vi "run_test_item.vi"(7 "DAQmx Device Name":tag="Dev1", 8 "error in":errorcluster, 10 "Test item":T2) -> (0 "error out":errorcluster, 1 "Test result":T1, 2 "Cluster":T6 {"Time Stamp" format="%<%.3X>T"})   [LabVIEW 2024]
doc: "The VI's input is a ctl_test_item_cluster. The output is the ctl_results_cluster indicator:\n- Time stamp: is the current time\n- Test item name: is the same as the Test item control's same label\n- Efficiency, Input Voltage, Output Voltage: pass criteria fulfilment for the measurement performed (perfrom_measurement.vi) based on the Test item.Stimuli cluster, results compared to the Test item.Pass limits cluster"
uses:
  OneDrive - Aalto University/SSIs - Semester 3/BME (1)/BME/vim report/dcdc_validator_project_Final (2)/dcdc_validator_project_Final/ctl_results_cluster.ctl
  OneDrive - Aalto University/SSIs - Semester 3/BME (1)/BME/vim report/dcdc_validator_project_Final (2)/dcdc_validator_project_Final/ctl_pass_fail_led.ctl
  OneDrive - Aalto University/SSIs - Semester 3/BME (1)/BME/vim report/dcdc_validator_project_Final (2)/dcdc_validator_project_Final/ctl_test_item_cluster.ctl
  OneDrive - Aalto University/SSIs - Semester 3/BME (1)/BME/vim report/dcdc_validator_project_Final (2)/dcdc_validator_project_Final/ctl_stimuli_cluster.ctl
  OneDrive - Aalto University/SSIs - Semester 3/BME (1)/BME/vim report/dcdc_validator_project_Final (2)/dcdc_validator_project_Final/ctl_loads_enum.ctl
  OneDrive - Aalto University/SSIs - Semester 3/BME (1)/BME/vim report/dcdc_validator_project_Final (2)/dcdc_validator_project_Final/ctl_pass_limits_cluster.ctl
  OneDrive - Aalto University/SSIs - Semester 3/BME (1)/BME/vim report/dcdc_validator_project_Final (2)/dcdc_validator_project_Final/ctl_test_outputs_cluster.ctl
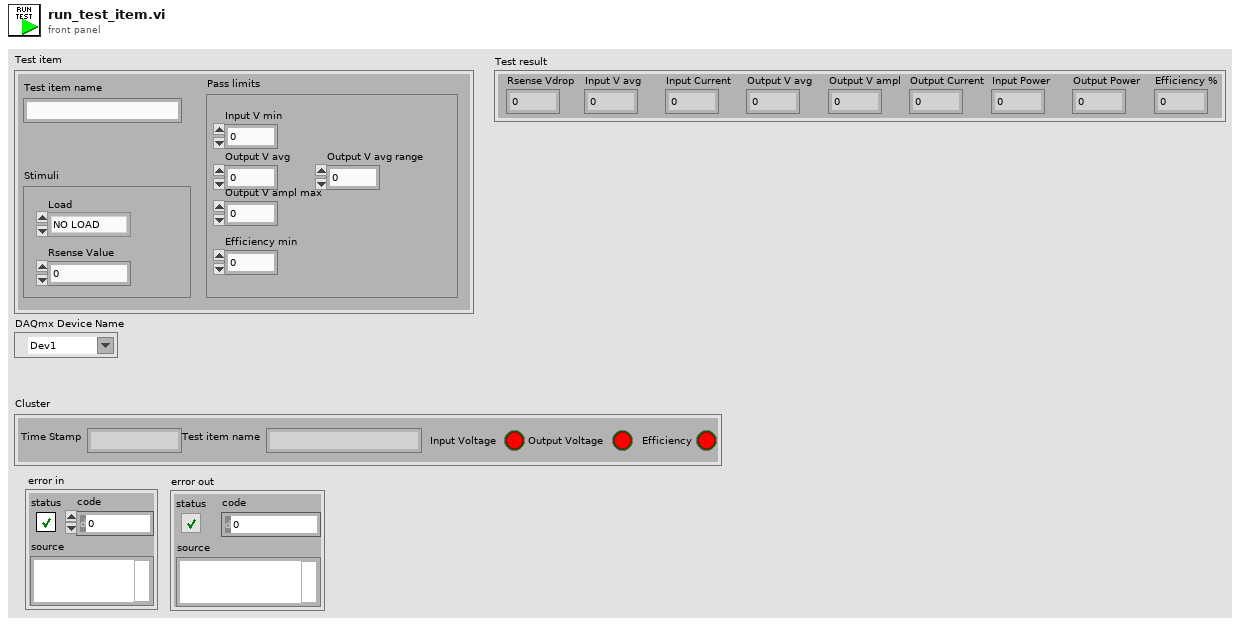
[diagram p1: front panel]
types:
  T1 = typedef "ctl_test_outputs_cluster.ctl" = cluster{"Output V avg":dbl, "Output V ampl":dbl, "Input Current":dbl, "Output Current":dbl, "Efficiency %":dbl, "Input V avg":dbl, "Input Power":dbl, "Output Power":dbl, "Rsense Vdrop":dbl}
  T2 = typedef "ctl_test_item_cluster.ctl" = cluster{"Stimuli":T3, "Pass limits":T5, "Test item name":string}
  T3 = typedef "ctl_stimuli_cluster.ctl" = cluster{"Load":T4, "Rsense Value":dbl}
  T4 = typedef "ctl_loads_enum.ctl" = enum16{"NO LOAD", "3.4", "4.7", "6.8", "2.8", "10", "1.6", "1.3", "3.2"}
  T5 = typedef "ctl_pass_limits_cluster.ctl" = cluster{"Output V avg":dbl, "Output V ampl max":dbl, "Efficiency min":dbl, "Input V min":dbl, "Output V avg range":dbl}
  T6 = typedef "ctl_results_cluster.ctl" = cluster{"Time Stamp":timestamp, "Test item name":string, "Input Voltage":T7, "Output Voltage":T7, "Efficiency":T7}
  T7 = typedef "ctl_pass_fail_led.ctl" = bool
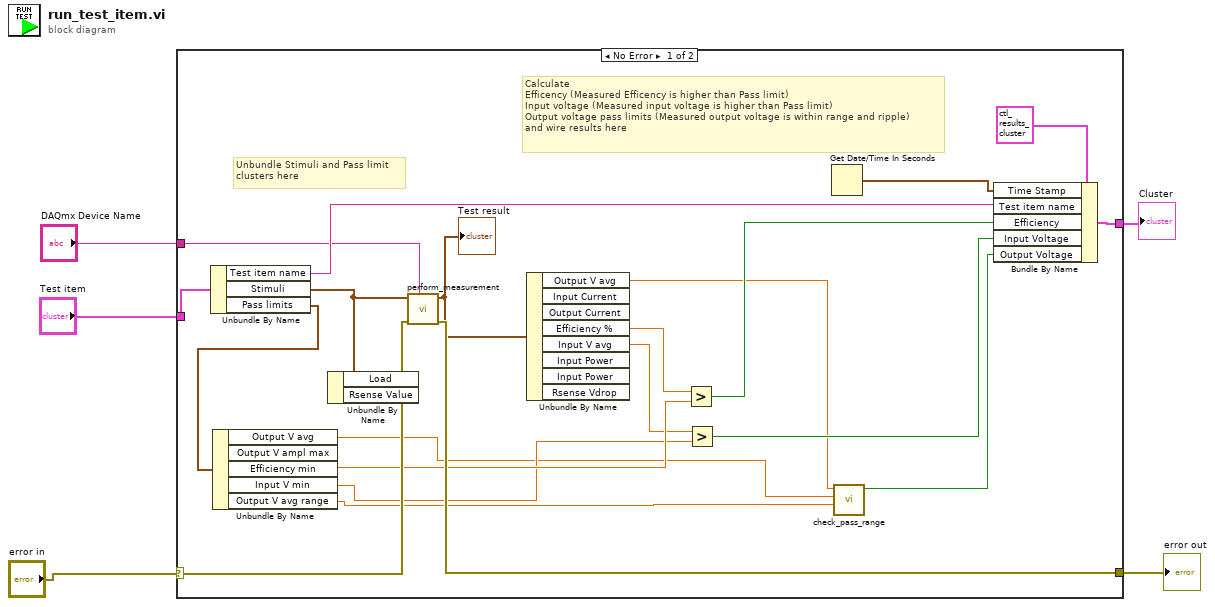
[diagram p0: block diagram]
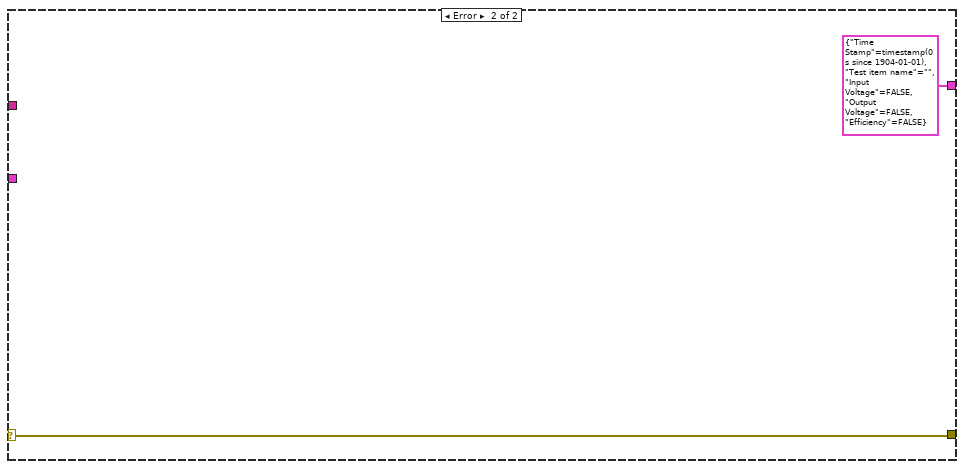
[diagram p2: hidden frame]
diagram:
  n1 = case shown="No Error" "error in" {
    selector: "error in" -> [w19 w28]
    tunnel: "Test item" -> [w26 _]
    tunnel: [w22 T6 {"Time Stamp"=timestamp(0 s since 1904-01-01), "Test item name"="", "Input Voltage"=FALSE, "Output Voltage"=FALSE, "Efficiency"=FALSE} ("Cluster")] -> w4
    tunnel: "DAQmx Device Name" -> [w21 _]
    tunnel: [w20 w28] -> w2
    frame No Error {
      # "Calculate\nEfficency (Measured Efficency is higher than Pass limit)\nInput voltage (Measured input voltage is higher than Pass limit)\nOutput voltage pass limits (Measured output voltage is within range and ripple)\nand wire results here"
      # "Unbundle Stimuli and Pass limit\nclusters here"
      n2 = Unbundle By Name(w26) -> ("Test item name"=w24:string, "Stimuli"=w18:T3, "Pass limits"=w17:T5)
      n3 = Unbundle By Name(w17) -> ("Output V avg"=w8:dbl, "Efficiency min"=w14:dbl, "Input V min"=w13:dbl, "Output V avg range"=w9:dbl)  [unwired: 1 out]
      n4 = Unbundle By Name(w18) -> ()  [unwired: 2 out]
      n5 = call "perform_measurement.vi"("DAQmx Device Name"=w21, "error in"=w19, "Stimuli"=w18) -> ("error out"=w20:errorcluster, "Outputs"=w16:T1)  [unwired: 6 in, 1 out]
      "Test result" <- w16
      n6 = Unbundle By Name(w16) -> ("Output V avg"=w7:dbl, "Efficiency %"=w15:dbl, "Input V avg"=w12:dbl)  [unwired: 5 out]
      n7 = Greater?(x=w15, y=w14) -> (0:w10:bool)
      n8 = Greater?(x=w12, y=w13) -> (0:w11:bool)
      n9 = Get Date/Time In Seconds() -> (seconds since 1Jan1904=w23:timestamp)
      n10 = call "check_pass_range.vi"("Output V avg range"=w9, "Output V avg center point"=w8, "Output V avg"=w7) -> ("Pass range?"=w6:bool)  [unwired: 8 in]
      n11 = Bundle By Name(cluster=T6 {"Time Stamp"=timestamp(0 s since 1904-01-01), "Test item name"="", "Input Voltage"=FALSE, "Output Voltage"=FALSE, "Efficiency"=FALSE} ("Cluster"), "Time Stamp"=w23, "Test item name"=w24, "Efficiency"=w10, "Input Voltage"=w11, "Output Voltage"=w6) -> (w22:T6)
    }
    frame Error {
    }
  }
  "Cluster" <- w4
  "error out" <- w2
